vi "avi_波形.vi"(8 "error in (no error)":errorcluster, 11 "Image":T1) -> (0 "error out":errorcluster, 2 "耗时":u32, 3 "波形":i32[](array[numeric]))   [LabVIEW 2017]
uses:
  <vilib>/vision/Image Controls.llb/IMAQ Image.ctl
panel:
  out "乘积;积;乘;product 2":i32
  out "乘积;积;乘;product":i32
  out "数组":i32[][](array[numeric])
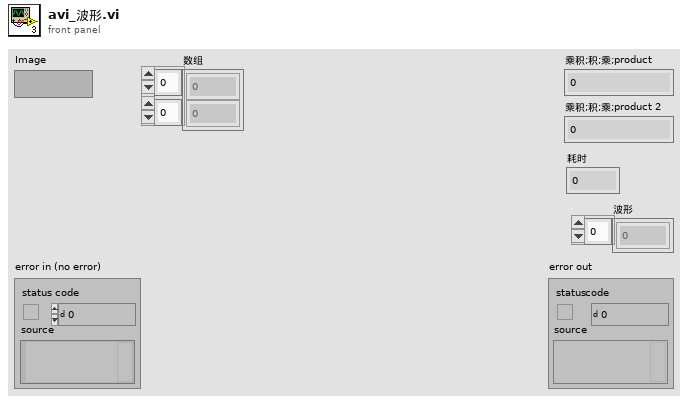
[diagram p1: front panel]
types:
  T1 = typedef "IMAQ Image.ctl" = refnum<image>
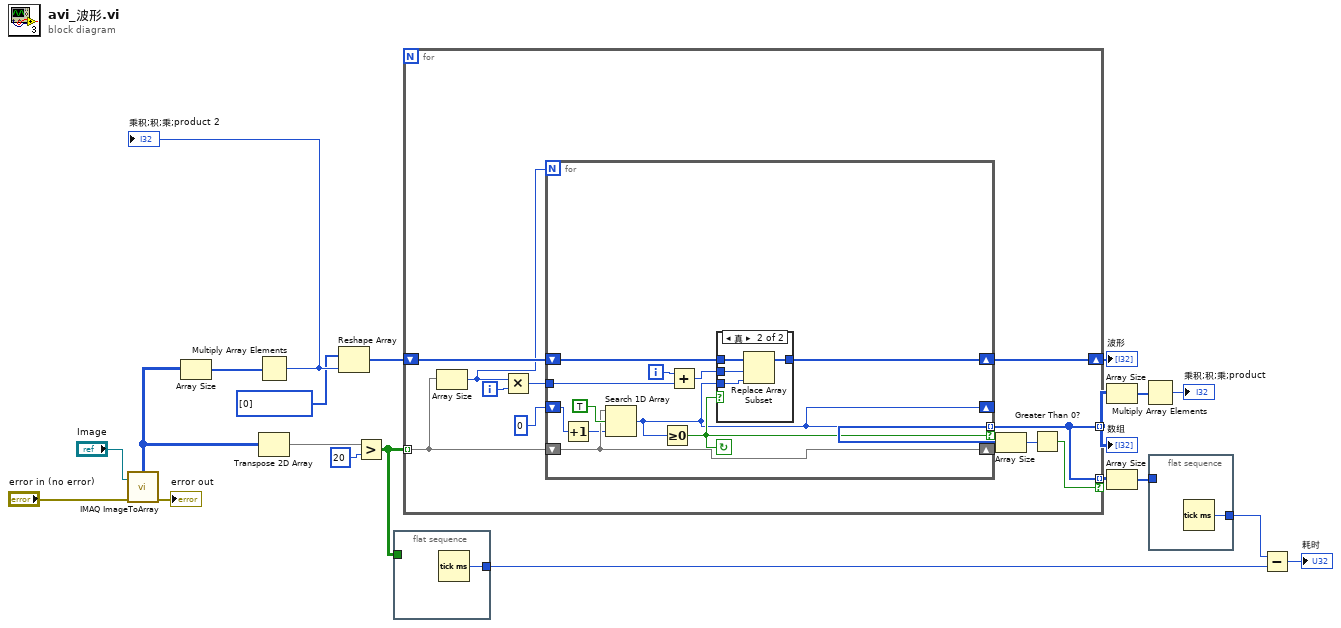
[diagram p0: block diagram]
diagram:
  n1 = call "IMAQ ImageToArray"("error in (no error)"="error in (no error)", "Image"="Image") -> ("error out"=→"error out":errorcluster, "Image Pixels (U8)"=w15:u8[][])  [unwired: 2 in, 3 out]
  n2 = Array Size(array=w15) -> (size(s)=w6:i32[])
  n3 = Multiply Array Elements(1:w6) -> (0:w5:i32)
  "乘积;积;乘;product 2" <- w5
  n4 = Transpose 2D Array(2D array=w15) -> (transposed array=w14:u8[][])
  n5 = Reshape Array(i32[] [0], w5) -> (w3:i32[])
  n6 = Greater?(x=w14, y=20) -> (0:w7:bool[][])
  n7 = flat-sequence {
    tunnel: w7 -> [_]
    tunnel: [w21] -> w11
    frame #0 {
      n8 = Tick Count (ms)() -> (millisecond timer value=w21:u32)
    }
  }
  n9 = for {
    tunnel: w7 -> [w30] mode=indexing
    tunnel: [w29] -> w16 mode=indexing
    tunnel: [w29] -> w9 mode=indexing if=w27
    shift-right: [w25] -> w2
    shift-left: w3 -> [w26]
    i -> [w23]
    n10 = Array Size(array=w30) -> (size(s)=w24:i32)
    n11 = Multiply(x=w24, y=w23) -> (x*y=w22:i32)
    n12 = for {
      N: w24 -> [_]
      shift-right: [w41] -> _
      shift-left: w30 -> [w41]
      shift-right: [w35] -> _
      shift-left: 0 ("index of element") -> [w40]
      tunnel: [w35] -> w29 mode=indexing if=w38
      shift-right: [w36] -> w25
      shift-left: w26 -> [w37]
      tunnel: w22 -> [w33]
      i -> [w34]
      stop <- w38 continue-if-true
      n13 = Increment(x=w40) -> (x+1=w39:i32)
      n14 = Search 1D Array(1D array=w41, element=TRUE ("元素"), start index (0)=w39) -> (index of element=w35:i32)
      n15 = Greater Or Equal To 0?(x=w35) -> (x >= 0?=w38:bool)
      n16 = Add(x=w34, y=w33) -> (x+y=w32:i32)
      n17 = case shown="真" w38 {
        tunnel: w37 -> [w43 w47]
        tunnel: [w43 w46] -> w36
        tunnel: w32 -> [_ w45]
        tunnel: w35 -> [_ w44]
        frame False {
        }
        frame True {
          n18 = Replace Array Subset(array=w47, new element=w44, index=w45) -> (w46:i32[])
        }
      }
    }
    n19 = Array Size(array=w29) -> (size(s)=w28:i32)
    n20 = Greater Than 0?(x=w28) -> (x > 0?=w27:bool)
  }
  "数组" <- w16
  "波形" <- w2
  n21 = Array Size(array=w16) -> (size(s)=w19:i32[])
  n22 = Array Size(array=w9) -> (size(s)=w8:i32[])
  n23 = Multiply Array Elements(1:w19) -> (0:→"乘积;积;乘;product":i32)
  n24 = flat-sequence {
    tunnel: [w48] -> w12
    tunnel: w8 -> [_]
    frame #0 {
      n25 = Tick Count (ms)() -> (millisecond timer value=w48:u32)
    }
  }
  n26 = Subtract(x=w12, y=w11) -> (x-y=→"耗时":u32)
